vi "RGB Pixels Values to Image.vi"(9 "I_RGB: Blue Color":u8[][](array[numeric]), 10 "I_RGB: Green Color":u8[][](array[numeric]), 11 "I_RGB: Red Color":u8[][](array[numeric])) -> (3 "O_Image Data":u8[](array[numeric]))   [LabVIEW 2015]
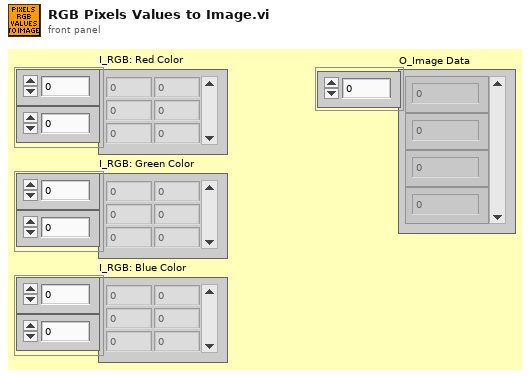
[diagram p1: front panel]
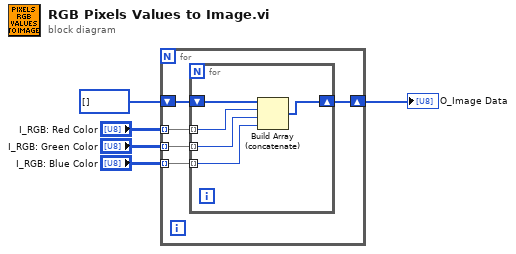
[diagram p0: block diagram]
diagram:
  n1 = for {
    tunnel: "I_RGB: Red Color" -> [w10] mode=indexing
    tunnel: "I_RGB: Green Color" -> [w9] mode=indexing
    tunnel: "I_RGB: Blue Color" -> [w8] mode=indexing
    shift-right: [w6] -> w1
    shift-left: u8[] [] ("appended array") -> [w7]
    n2 = for {
      tunnel: w10 -> [w15] mode=indexing
      tunnel: w9 -> [w14] mode=indexing
      tunnel: w8 -> [w13] mode=indexing
      shift-right: [w11] -> w6
      shift-left: w7 -> [w12]
      n3 = Build Array (concatenate)(w12, w15, w14, w13) -> (w11:u8[])
    }
  }
  "O_Image Data" <- w1
